vi "read_green_level.vi"(0 "error in":errorcluster, 3 "node":string) -> (1 "error out":errorcluster, 4 "green level":ext)   [LabVIEW 2015]
doc: "Reads green light level"
uses:
  ROS/Code/Console/Servers/ServerSubs/TopicDef.ctl
  ROS/Code/SubVIs/_ROSDirection.ctl
  ROS/MessageParsing/std_msgs/subs/parse_float32_scalar.vi
panel:
  out "Reply":string
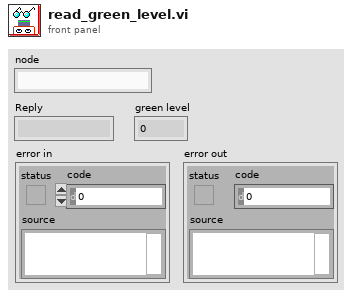
[diagram p1: front panel]
types:
  T1 = typedef "TopicDef.ctl" = cluster{"Topic":string, "Type":string, "Action":T2, "Update (ms)":u16, "queue size":u16}
  T2 = typedef "_ROSDirection.ctl" = enum16{"Node", "Publisher", "Subscriber", "ServiceClient", "ServiceProvider"}
  T3 = typedef "_ROSControl.ctl" = cluster{"topic port":u16, "Node":string, "topic":string, "type":string, "node port":u16, "error ":errorcluster, "Direction":T2, "Update (ms)":u16, "FIFO size":u16}
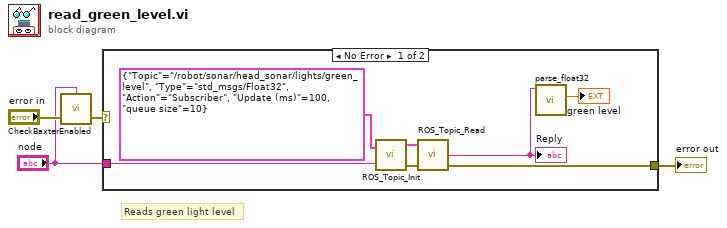
[diagram p0: block diagram]
diagram:
  # "Reads green light level"
  n1 = call "CheckBaxterEnabled.vi"("error in"="error in", "node"="node") -> ("error out"=w3:errorcluster)  [unwired: 2 in]
  n2 = case shown="No Error" w3 {
    selector: w3 -> [_ w12]
    tunnel: "node" -> [w11 _]
    tunnel: [w7 w12] -> w1
    frame No Error {
      n3 = call "ROS_Topic_Init.vi"("Definitions"=T1 {"Topic"="/robot/sonar/head_sonar/lights/green_level", "Type"="std_msgs/Float32", "Action"=enum."Subscriber", "Update (ms)"=100, "queue size"=10}, "node"=w11) -> ("ROS out"=w9:T3, "error out"=w8:errorcluster)  [unwired: 1 in]
      n4 = call "ROS_Topic_Read.vi"("error in (no error)"=w8, "ROS in"=w9) -> ("error out"=w7:errorcluster, "Reply"=w6:string)  [unwired: 1 in, 1 out]
      "Reply" <- w6
      n5 = call-poly "parse_float32.vi"("msg in"=w6) -> ("number"=→"green level":sgl)  [unwired: 4 in, 2 out]
    }
    frame Error {
    }
  }
  "error out" <- w1
